vi "Logging Write Loop.vi"(4 "Delay":u32=50, 5 "LoggingDevRef":T1) -> ()   [LabVIEW 2012, in "femtoRoboLib.lvlib"]
uses:
  femtoRoboLib.lvlib
  LoggingDevRef.ctl
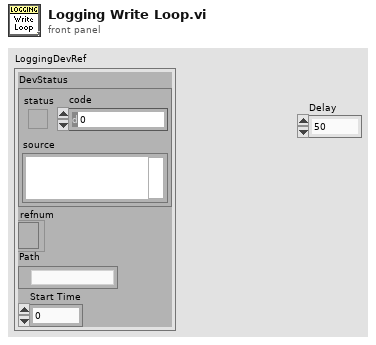
[diagram p1: front panel]
types:
  T1 = typedef "femtoRoboLib.lvlib/LoggingDevRef.ctl" = cluster{"DevStatus":errorcluster, "refnum":refnum<file>, "Path":path, "Start Time":u32}
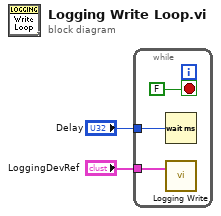
[diagram p0: block diagram]
diagram:
  n1 = while {
    tunnel: "LoggingDevRef" -> [w5]
    tunnel: "Delay" -> [w4]
    stop <- FALSE stop-if-true
    n2 = Wait (ms)(milliseconds to wait=w4) -> ()  [unwired: 1 out]
    n3 = call "Logging Write.vi"("LoggingDevRef"=w5) -> ()  [unwired: 2 in, 3 out]
  }
